vi "Tosca-Setup General Options.vi"(5 "Options In":T1) -> (6 "Options Out":T1, 8 "Canceled?":bool)   [LabVIEW 2020]
uses:
  epl-vi-lib/Utility VIs/Buttons/KCheckmarkBoolean 2.ctl
  Typedefs/Tosca-General Options.ctl
panel:
  in  "DI dt":i32=1 caption="Digital input resolution (ms)" min=1
  in  "headway":dbl=1.0 caption="AO headway (%)" min=0.0 max=200.0 step=1.0
  in  "max errors":i32=1 caption="Quit after this many errors" min=1
  in  "AutoDI":T2 caption="Automatically start digital input"
  in  "Cancel":bool
  in  "Apply":bool
  # "Options"
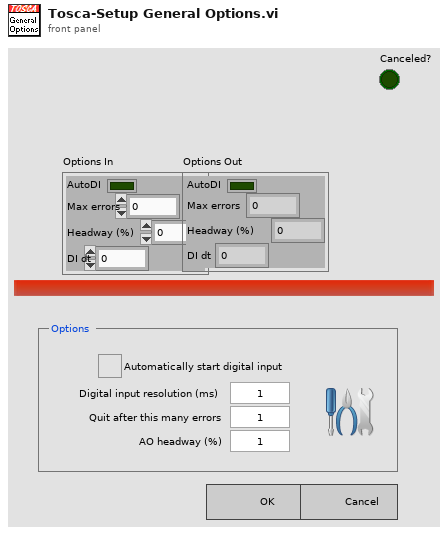
[diagram p1: front panel]
types:
  T1 = typedef "Tosca-General Options.ctl" = cluster{"AutoDI":bool, "Max errors":i32, "Headway (%)":dbl, "DI dt":i32}
  T2 = typedef "KCheckmarkBoolean 2.ctl" = bool
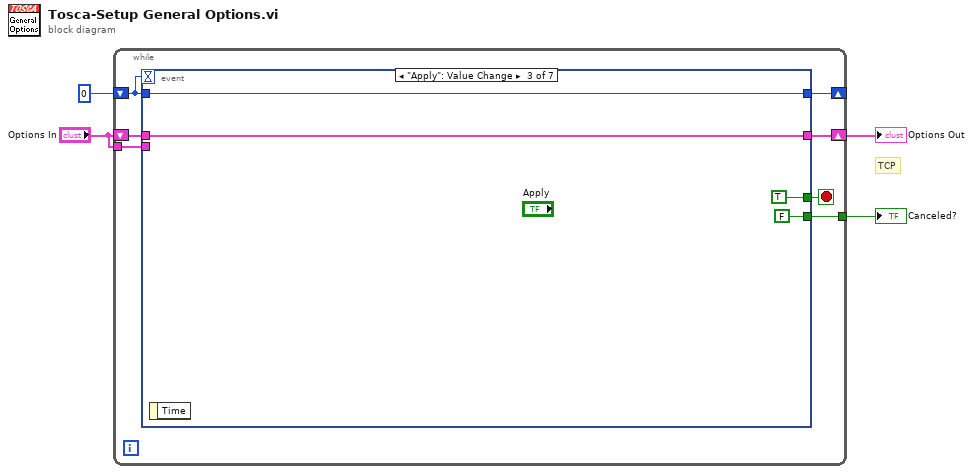
[diagram p0: block diagram]
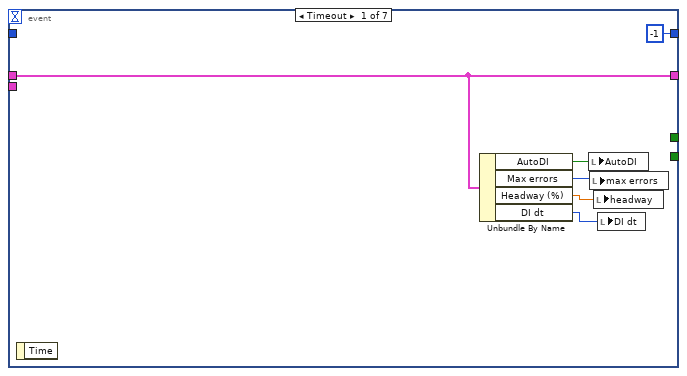
[diagram p2: hidden frame]
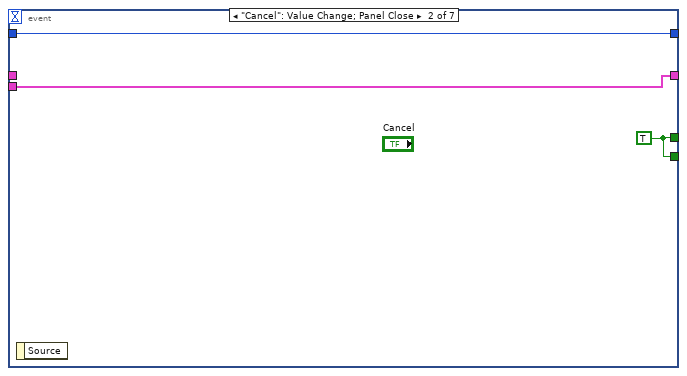
[diagram p3: hidden frame]
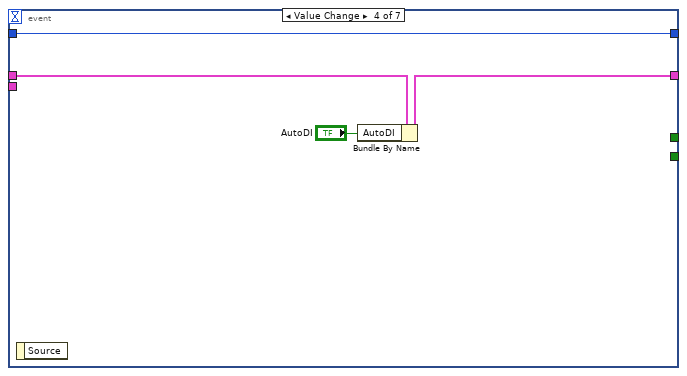
[diagram p4: hidden frame]
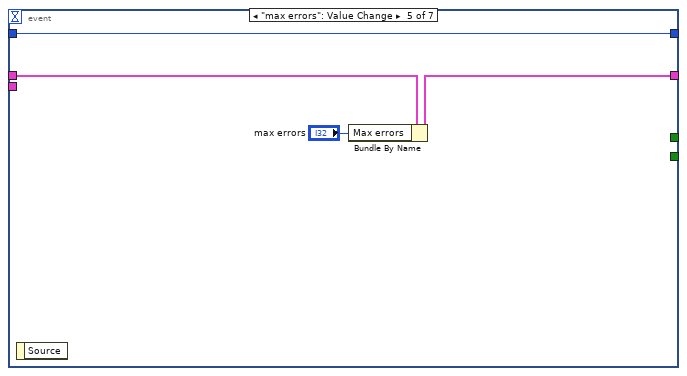
[diagram p5: hidden frame]
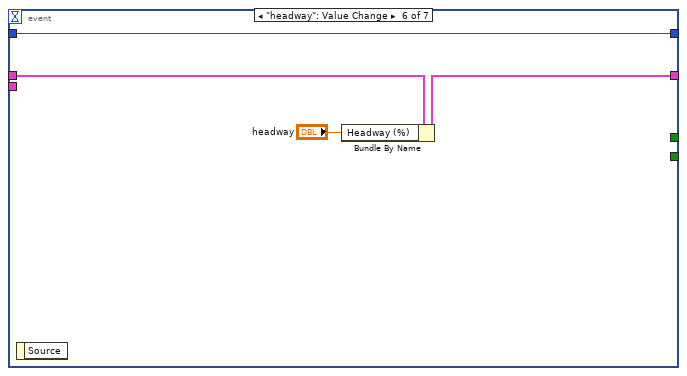
[diagram p6: hidden frame]
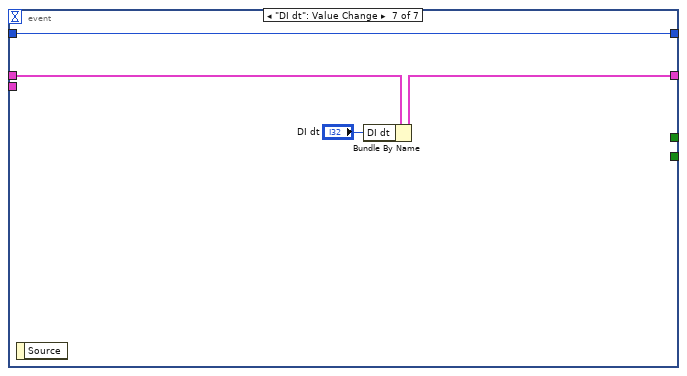
[diagram p7: hidden frame]
diagram:
  # "TCP"
  n1 = while {
    shift-right: [w11] -> _
    shift-left: 0 -> [w5]
    tunnel: [w9] -> w3
    tunnel: "Options In" -> [w6]
    shift-right: [w7] -> w1
    shift-left: "Options In" -> [w8]
    stop <- w10 stop-if-true
    n2 = event shown="[2] \"Apply\": Value Change" {
      selector: _ -> [_ _ _ _ _ _ _]
      dyn-events: _ -> [_ _ _ _ _ _ _]
      timeout: w5 -> [_ _ _ _ _ _ _]
      tunnel: [-1 w18 w21 w27 w31 w35 w39] -> w11
      tunnel: [_ w20 TRUE _ _ _ _] -> w10
      tunnel: [_ w20 FALSE _ _ _ _] -> w9
      tunnel: w8 -> [w16 _ w22 w28 w32 w36 w40]
      tunnel: [w16 w19 w22 w26 w30 w34 w38] -> w7
      tunnel: w6 -> [_ w19 _ _ _ _ _]
      tunnel: w5 -> [_ w18 w21 w27 w31 w35 w39]
      event Timeout {
        n3 = event-data() -> ()  [unwired: 1 in, 1 out]
        n4 = Unbundle By Name(w16) -> ("AutoDI"=w15:bool, "Max errors"=w14:i32, "Headway (%)"=w13:dbl, "DI dt"=w12:i32)
        n5 = local write "AutoDI"(w15) -> ()
        n6 = local write "max errors"(w14) -> ()
        n7 = local write "headway"(w13) -> ()
        n8 = local write "DI dt"(w12) -> ()
      }
      event "Cancel": Value Change; Panel Close {
        w20 = TRUE
        n9 = event-data() -> ()  [unwired: 1 in, 1 out]
      }
      event "Apply": Value Change {
        n10 = event-data() -> ()  [unwired: 1 in, 1 out]
      }
      event Value Change {
        n11 = event-data() -> ()  [unwired: 1 in, 1 out]
        n12 = Bundle By Name(cluster=w28, "AutoDI"="AutoDI") -> (w26:T1)
      }
      event "max errors": Value Change {
        n13 = event-data() -> ()  [unwired: 1 in, 1 out]
        n14 = Bundle By Name(cluster=w32, "Max errors"="max errors") -> (w30:T1)
      }
      event "headway": Value Change {
        n15 = event-data() -> ()  [unwired: 1 in, 1 out]
        n16 = Bundle By Name(cluster=w36, "Headway (%)"="headway") -> (w34:T1)
      }
      event "DI dt": Value Change {
        n17 = event-data() -> ()  [unwired: 1 in, 1 out]
        n18 = Bundle By Name(cluster=w40, "DI dt"="DI dt") -> (w38:T1)
      }
    }
  }
  "Canceled?" <- w3
  "Options Out" <- w1
